vi "Generate Trace for New Actor.vi"(8 "Debug Alias":string, 9 "Class Name":string, 10 "Actor Enqueuer":refnum<class "Message Enqueuer.lvclass">, 11 "Caller Enqueuer":refnum<class "Message Enqueuer.lvclass">) -> ()   [LabVIEW 2020, in "AF Debug.lvlib"]
doc: "Generates a DETT User Generated Trace for an actor being newly launched."
uses:
  AF Debug.lvlib
  Register Actor Msg/Register Actor Msg.lvclass
  Registration Mode.ctl
  Localized Strings.vi
  ActorFramework/Message Enqueuer/Message Enqueuer.lvclass
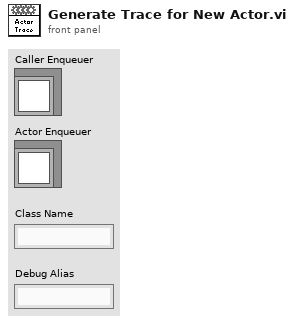
[diagram p1: front panel]
types:
  T1 = typedef "AF Debug.lvlib/Registration Mode.ctl" = enum16{"Register Actor", "Get ID", "Get Enqueuer", "Deregister Actor", "Get Update Event", "Get All Actors"}
  T2 = typedef "AF Debug.lvlib/This Actor.ctl" = cluster{"Enqueuer":refnum<class "Message Enqueuer.lvclass">, "ID":string, "Alias":string, "Actor Core Name":string, "Details":cluster{"Qualified Name":string, "Caller ID":string}}
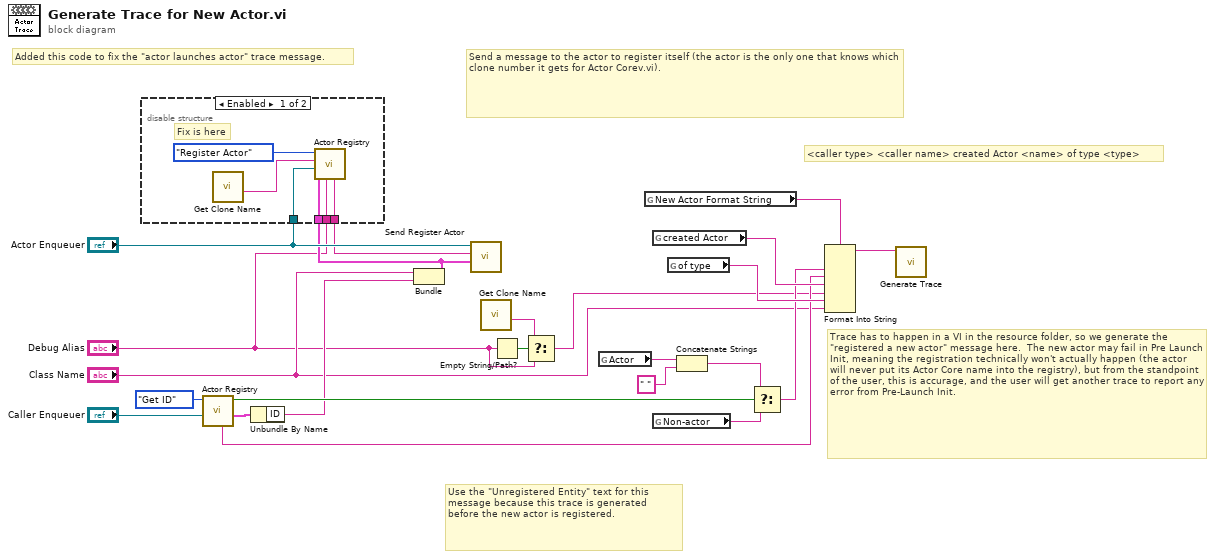
[diagram p0: block diagram]
diagram:
  # "Added this code to fix the \"actor launches actor\" trace message."
  # "Use the \"Unregistered Entity\" text for this message because this trace is generated before the new actor is registered."
  # "Trace has to happen in a VI in the resource folder, so we generate the \"registered a new actor\" message here.  The new actor may fail in Pre Launch Init, meaning the registration technically won't actually happen (the actor will never put its Actor Core name into the registry), but from the standpoint of the user, this is accurage, and the user will get another trace to report any error from Pre-Launch Init."
  # "<caller type> <caller name> created Actor <name> of type <type>"
  # "Send a message to the actor to register itself (the actor is the only one that knows which clone number it gets for Actor Corev.vi)."
  n1 = call "Actor Registry.vi"("Actor Enqueuer"="Caller Enqueuer", "Action"=Registration_Mode."Get ID") -> ("This Actor"=w23:T2, "Found"=w11:bool, "Actor Alias out"=w10:string)  [unwired: 5 in, 2 out]
  n2 = Unbundle By Name(w23) -> ("ID"=w9:string)
  n3 = Bundle("Class Name"="Class Name", "ID"=w9) -> (w3:cluster{"Class Name":string, "ID":string})  [unwired: 1 in]
  n4 = disable-structure shown="Enabled" {
    disable-tunnel: "Actor Enqueuer" -> [w28 _]
    disable-tunnel: w3 -> [w27 _]
    disable-tunnel: "Debug Alias" -> [w26 w30]
    disable-tunnel: [w25 w30] -> w1
    frame Enabled {
      # "Fix is here"
      n5 = call "Get Clone Name.vi"() -> ("Clone ID"=w24:string)  [unwired: 10 in, 1 out]
      n6 = call "Actor Registry.vi"("Actor Alias"=w26, "Details"=w27, "Actor Enqueuer"=w28, "Actor ID"=w24, "Action"=Registration_Mode."Register Actor") -> ("Actor Alias out"=w25:string)  [unwired: 2 in, 4 out]
    }
    frame Disabled {
      # "Original code"
    }
  }
  n7 = call "Send Register Actor.vi"("Details"=w3, "Debug Alias"=w1, "Message Enqueuer"="Actor Enqueuer") -> ()  [unwired: 7 in, 2 out]
  n8 = call "Get Clone Name.vi"() -> ("Clone ID"=w5:string)  [unwired: 10 in, 1 out]
  n9 = Empty String/Path?(string/path="Debug Alias") -> (empty?=w8:bool)
  n10 = Select(t=w5, s=w8, f="Debug Alias") -> (s? t:f=w6:string)
  n11 = global read "Localized Strings.vi" "Actor"() -> (w17:string)
  n12 = global read "Localized Strings.vi" "New Actor Format String"() -> (w13:string)
  n13 = global read "Localized Strings.vi" "created Actor"() -> (w14:string)
  n14 = global read "Localized Strings.vi" "Non-actor"() -> (w16:string)
  n15 = global read "Localized Strings.vi" "of type"() -> (w15:string)
  n16 = Concatenate Strings(w17, " " ("string")) -> (w18:string)
  n17 = Select(t=w18, s=w11, f=w16) -> (s? t:f=w12:string)
  n18 = Format Into String(format string=w13, w12, w10, w14, w6, w15, "Class Name") -> (resulting string=w20:string)  [unwired: 2 in, 1 out]
  n19 = call "Generate Trace.vi"("String"=w20) -> ()  [unwired: 11 in]
